vi "Write 7z config.vi"(8 "error in (no error)":errorcluster, 11 "PostBuildSupport in":refnum<class "PostBuildSupport.lvclass">) -> (0 "error out":errorcluster, 3 "PostBuildSupport out":refnum<class "PostBuildSupport.lvclass">)   [LabVIEW 2016, in "PostBuildSupport.lvclass"]
uses:
  PostBuildSupport.lvclass
  PostBuildSupport.lvclass/PostBuildSupport.ctl
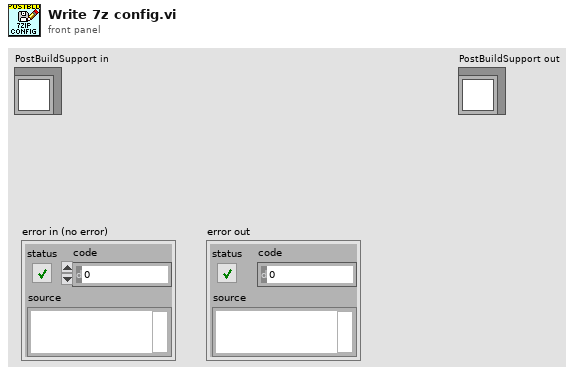
[diagram p1: front panel]
types:
  T1 = enum16{"open", "replace", "create", "open or create", "replace or create", "replace or create with confirmation"}
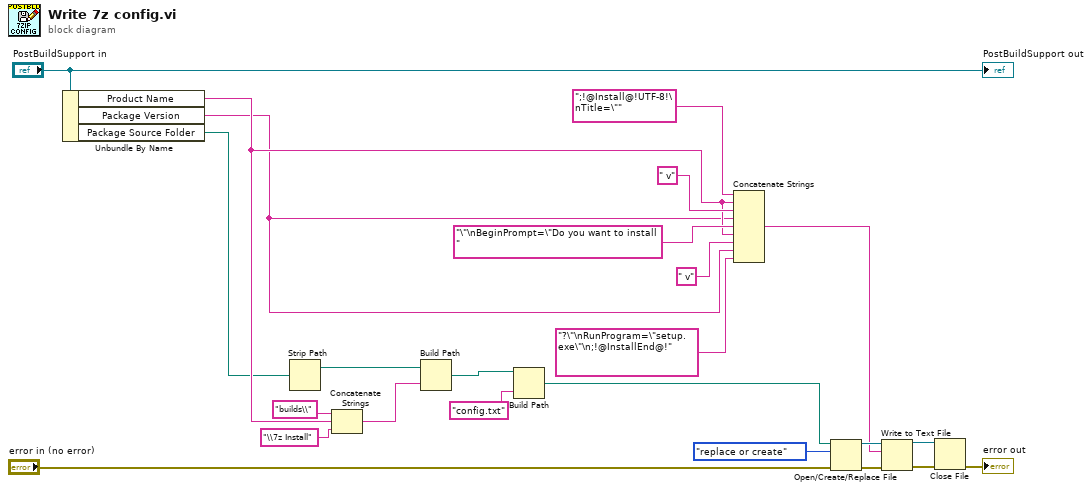
[diagram p0: block diagram]
diagram:
  n1 = Unbundle By Name("PostBuildSupport in") -> ("Product Name"=w3:string, "Package Version"=w1:string, "Package Source Folder"=w2:path)
  n2 = Strip Path(path=w2) -> (stripped path=w23:path)  [unwired: 1 out]
  n3 = Concatenate Strings("builds\\" ("name or relative path"), w3, "\\7z Install" ("name or relative path")) -> (w5:string)
  n4 = Build Path(base path=w23, name or relative path=w5) -> (appended path=w12:path)
  n5 = Build Path(base path=w12, name or relative path="config.txt") -> (appended path=w17:path)
  n6 = Concatenate Strings(";!@Install@!UTF-8!\nTitle=\"" ("Name of target (My Computer)"), w3, " v" ("Name of target (My Computer)"), w1, "\"\nBeginPrompt=\"Do you want to install " ("Name of target (My Computer)"), w3, " v" ("Name of target (My Computer)"), w1, "?\"\nRunProgram=\"setup.exe\"\n;!@InstallEnd@!" ("Name of target (My Computer)")) -> (w20:string)
  n7 = Open/Create/Replace File(file path (use dialog)=w17, error in="error in (no error)", operation (0:open)=T1."replace or create") -> (refnum out=w21:refnum<file>, error out=w18:errorcluster)  [unwired: 3 in, 1 out]
  n8 = Write to Text File(file (use dialog)=w21, text=w20, error in=w18) -> (refnum out=w14:refnum<file>, error out=w15:errorcluster)  [unwired: 1 in, 1 out]
  n9 = Close File(refnum=w14, error in=w15) -> (error out=→"error out":errorcluster)  [unwired: 1 out]
  "PostBuildSupport out" <- "PostBuildSupport in"
